vi "Report.vi"(4 "GuiRef":T1={"StringOut"=refnum, "AbortOnFail"=refnum, "SN"=refnum, "SN_Length"=refnum, "TestResult"=refnum, "Starttime"=refnum, "CycleTime"=refnum, "ErrorCode"=refnum, "UUTStatus"=refnum, "DataBaseEnable?"=refnum, "DUTModel"=refnum, "FixtureID"=refnum, "OperatorID"=refnum, "SNReady"=refnum, "StopSlot"=refnum, "NextStep"=refnum, "SlotStart?"=refnum, "PassYeild"=refnum, "Failed"=refnum, "Passed"=refnum, "Tested"=refnum, "ErrorStop"=refnum, "SlotReady"=refnum, "StartTest"=refnum, "TestItemsCtl"={"StepName"="", "TestEnable"=FALSE, "LoopCount"=0, "StopOnFail"=FALSE, "LastStep?"=FALSE, "Index"=0, "Para1"="", "Para2"="", "Para3"="", "Para4"="", "Para5"="", "TimeStart"=0}, "ProcessBar"=refnum, "Slot"=enum."Slot1", "Row"=3, "States"=refnum, "TestMode"=refnum, "PassYeild"=refnum, "ShowSkipStep?"=FALSE, "IniConfig"=refnum, "循环次数-DUT"=refnum, "开始按钮-DUT"=refnum, "选择方式"=refnum, "ExcelNames"=refnum, "TestPara"=refnum, "DAQmx设备名"=refnum, "波形图"=refnum, "调试模式"=refnum, "输入电压"=refnum, "产品型号"=refnum, "上电"=refnum, "测试结果"=refnum, "测试项目"=refnum, "DAQConfig"=refnum}, 5 "Report":string[][](array[string]), 6 "TestConfig":string[][](array[string]), 7 "索引":i32=2, 8 "index":i32=3, 9 "FailStep":string="XXX", 10 "TestResult":bool, 11 "TestStep":string="小灯") -> (3 "ReportOut":string[][](array[string]))   [LabVIEW 2013]
uses:
  SystemCode/Subvi/RefToString.vi
  <vilib>/Utility/miscctls.llb/LVRowAndColumnUnsignedTypeDef.ctl
  SystemCode/SysControl/TestItemsCTL.ctl
  SystemCode/SysControl/Slot.ctl
  SystemCode/SysControl/Reference.ctl
panel:
  out "StepReport":string[](array[string])
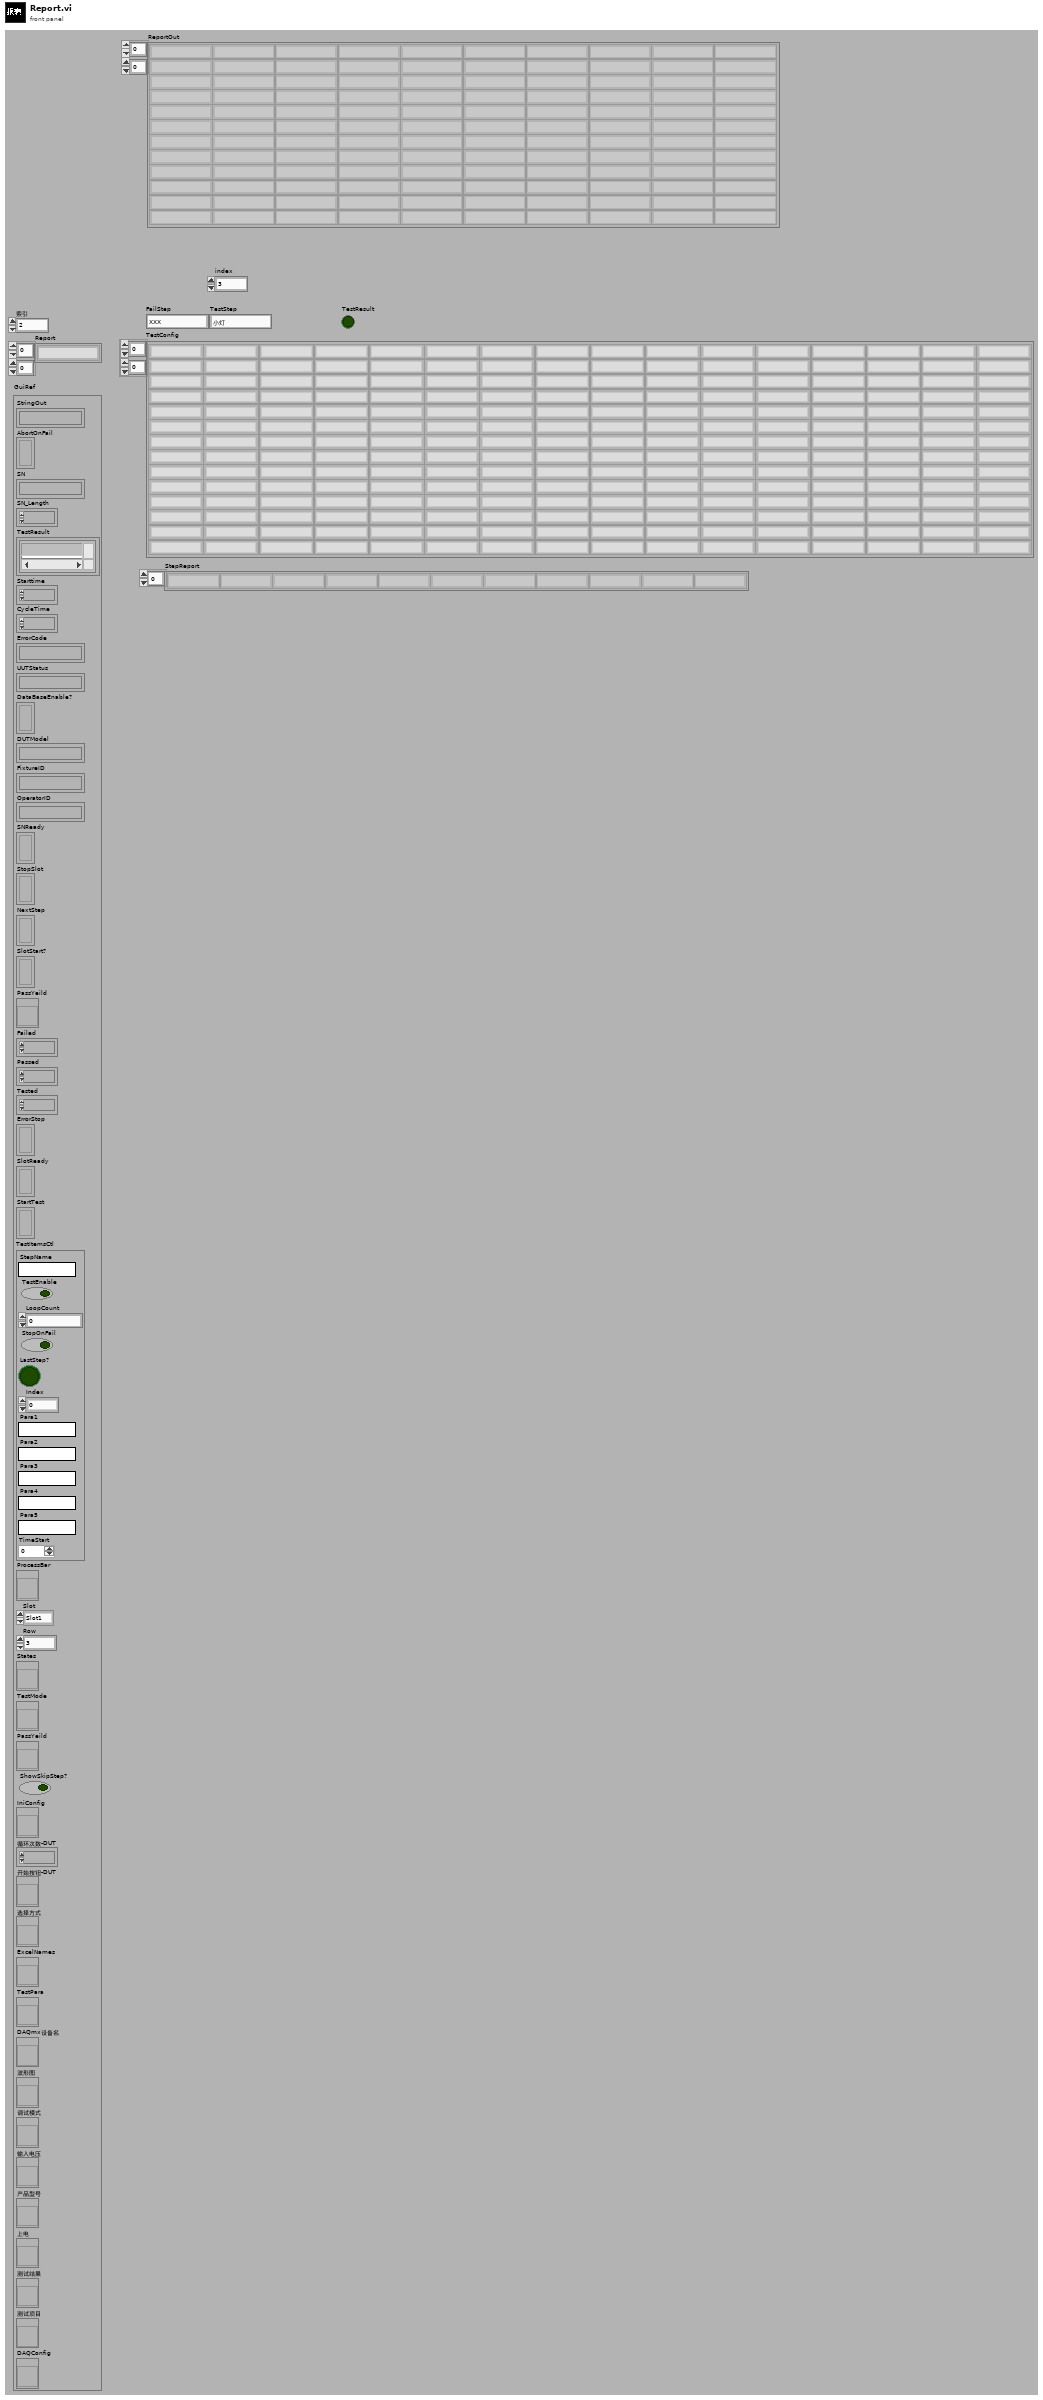
[diagram p1: front panel]
types:
  T1 = typedef "Reference.ctl" = cluster{"StringOut":refnum<vi>, "AbortOnFail":refnum<vi>, "SN":refnum<vi>, "SN_Length":refnum<vi>, "TestResult":refnum<vi>, "Starttime":refnum<vi>, "CycleTime":refnum<vi>, "ErrorCode":refnum<vi>, "UUTStatus":refnum<vi>, "DataBaseEnable?":refnum<vi>, "DUTModel":refnum<vi>, "FixtureID":refnum<vi>, "OperatorID":refnum<vi>, "SNReady":refnum<vi>, "StopSlot":refnum<vi>, "NextStep":refnum<vi>, "SlotStart?":refnum<vi>, "PassYeild":refnum<vi>, "Failed":refnum<vi>, "Passed":refnum<vi>, "Tested":refnum<vi>, "ErrorStop":refnum<vi>, "SlotReady":refnum<vi>, "StartTest":refnum<vi>, "TestItemsCtl":T2, "ProcessBar":refnum<vi>, "Slot":T3, "Row":i32, "States":refnum<vi>, "TestMode":refnum<vi>, "PassYeild":refnum<vi>, "ShowSkipStep?":bool, "IniConfig":refnum<vi>, "循环次数-DUT":refnum<vi>, "开始按钮-DUT":refnum<vi>, "选择方式":refnum<vi>, "ExcelNames":refnum<vi>, "TestPara":refnum<vi>, "DAQmx设备名":refnum<vi>, "波形图":refnum<vi>, "调试模式":refnum<vi>, "输入电压":refnum<vi>, "产品型号":refnum<vi>, "上电":refnum<vi>, "测试结果":refnum<vi>, "测试项目":refnum<vi>, "DAQConfig":refnum<vi>}
  T2 = typedef "TestItemsCTL.ctl" = cluster{"StepName":string, "TestEnable":bool, "LoopCount":i32, "StopOnFail":bool, "LastStep?":bool, "Index":i32, "Para1":string, "Para2":string, "Para3":string, "Para4":string, "Para5":string, "TimeStart":u32}
  T3 = typedef "Slot.ctl" = enum16{"Slot1", "Slot2", "Slot3", "Slot4"}
  T4 = typedef "LVRowAndColumnUnsignedTypeDef.ctl" = cluster{"Row":u32, "Column":u32}
  T5 = enum32{"invalid app kind", "Development System", "Run Time System", "Student Edition", "Embedded LabVIEW", "Evaluation", "Custom"}
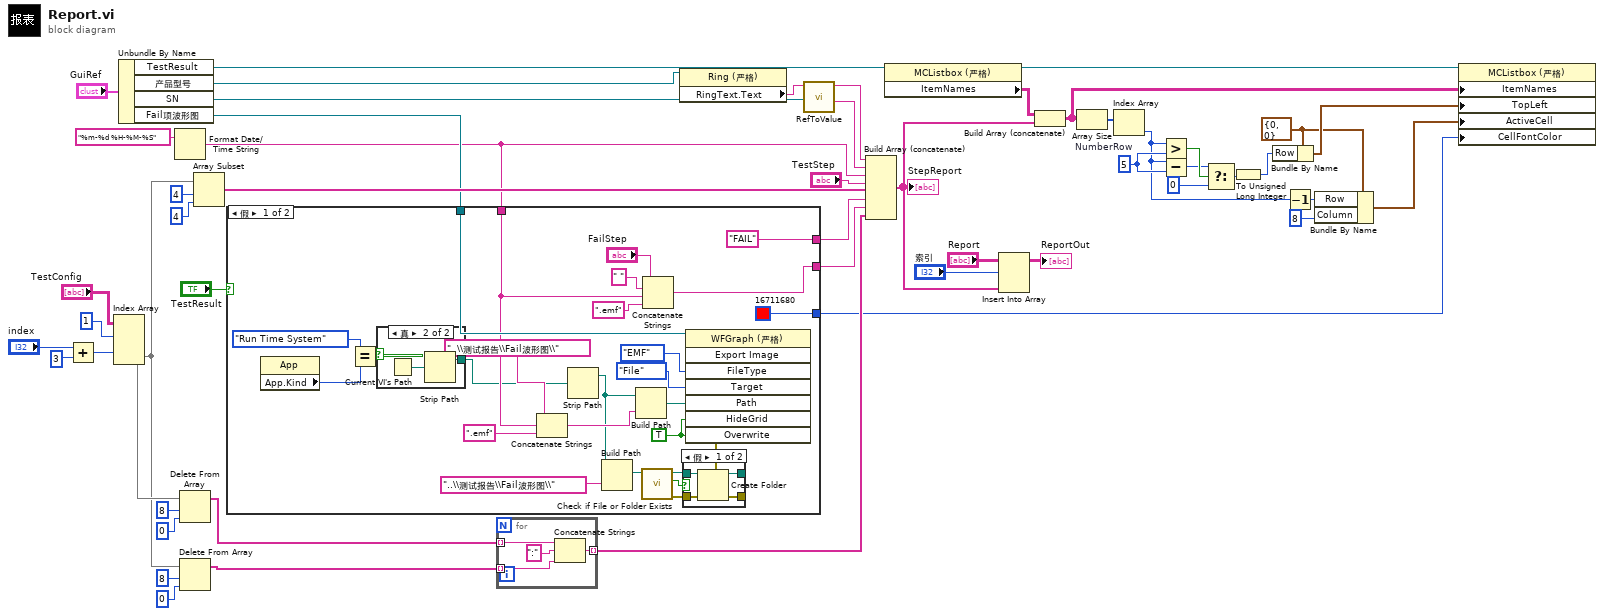
[diagram p0: block diagram]
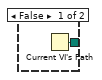
[diagram p3: hidden frame]
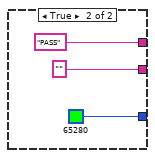
[diagram p4: hidden frame]
diagram:
  w4 = T4 {"Row"=0, "Column"=0} ("Top Left Visible Cell")
  w28 = 5  # NumberRow
  n1 = Add(x="index", y=3) -> (x+y=w33:i32)
  n2 = Index Array(array="TestConfig", index (row) #1=1 ("索引 (行)"), index (row) #2=w33) -> (element #1=w47:string[], element #2=w19:string[])  [unwired: 2 in]
  n3 = Unbundle By Name("GuiRef") -> ("TestResult"=w16:refnum<vi>, "产品型号"=w10:refnum<vi>, "SN"=w31:refnum<vi>, "Fail项波形图"=w18:refnum<vi>)
  n4 = Format Date/Time String(time format string (%c)="%m-%d %H-%M-%S" ("时间格式字符串(%c)")) -> (date/time string=w17:string)  [unwired: 2 in]
  n5 = Delete From Array(array=w47, length=8 ("长度"), index=0 ("索引")) -> (array with subset deleted=w46:string[])  [unwired: 1 out]
  n6 = Delete From Array(array=w19, length=8 ("长度"), index=0 ("索引")) -> (array with subset deleted=w45:string[])  [unwired: 1 out]
  n7 = Array Subset(array=w19, index=4 ("索引"), length=4 ("长度")) -> (w40:string[])
  n8 = case shown="假" "TestResult" {
    tunnel: ["FAIL" ("元素") "PASS" ("元素")] -> w37
    tunnel: [w67 "" ("FailStep")] -> w36
    tunnel: w18 -> [w72 _]
    tunnel: w17 -> [w68 _]
    tunnel: [u32 16711680 u32 65280] -> w5
    frame False {
      w73 = TRUE ("始终覆盖")
      n9 = property class="App"() -> ("App.Kind"=w62:T5)  [unwired: 2 in, 2 out]
      n10 = Equal?(x=T5."Run Time System" ("y"), y=w62) -> (x = y?=w61:bool)
      n11 = case shown="真" w61 {
        tunnel: [w83 w85] -> w60
        frame False {
          n12 = Current VI's Path() -> (path=w83:path)
        }
        frame True {
          n13 = Current VI's Path() -> (path=w84:path)
          n14 = Strip Path(path=w84) -> (stripped path=w85:path)  [unwired: 1 out]
        }
      }
      n15 = Concatenate Strings("..\\测试报告\\Fail波形图\\" ("字符串"), w68, ".emf" ("字符串")) -> (w65:string)
      n16 = Strip Path(path=w60) -> (stripped path=w58:path)  [unwired: 1 out]
      n17 = Build Path(base path=w58, name or relative path="..\\测试报告\\Fail波形图\\" ("字符串")) -> (appended path=w57:path)
      n18 = Build Path(base path=w58, name or relative path=w65) -> (appended path=w64:path)
      n19 = call <vilib>:"Check if File or Folder Exists.vi"("path"=w57) -> ("error out"=w54:errorcluster, "file or folder exists?"=w55:bool, "dup path"=w56:path)  [unwired: 1 in, 7 out]
      n20 = Concatenate Strings("FailStep", " " ("字符串"), w68, ".emf" ("字符串")) -> (w67:string)
      n21 = case shown="假" w55 {
        tunnel: w56 -> [w81 w82]
        tunnel: [w80 _] -> w53
        tunnel: w54 -> [w79 _]
        tunnel: [w78 w82] -> _
        frame False {
          n22 = Create Folder(path (use dialog)=w81, error in=w79) -> (created path=w78:path, error out=w80:errorcluster)  [unwired: 2 out]
        }
        frame True {
        }
      }
      n23 = invoke on="调用节点" class="WFGraph (严格)" method="Export Image"(reference=w72, error in=w53, "FileType"=enum32{"BMP", "EPS", "EMF", "PICT"}."EMF" ("文件类型"), "Target"=enum32{"File", "Clipboard"}."File" ("终端"), "Path"=w64, "HideGrid"=w73, "Overwrite"=w73) -> ()  [unwired: 1 in, 8 out]
    }
    frame True {
    }
  }
  n24 = for {
    tunnel: w46 -> [w92] mode=indexing
    tunnel: w45 -> [w91] mode=indexing
    tunnel: [w89] -> w39 mode=indexing
    n25 = Concatenate Strings(w92, ":" ("字符串"), w91) -> (w89:string)
  }
  n26 = property class="Ring (严格)"(reference=w10) -> ("RingText.Text"=w9:string)  [unwired: 1 in, 2 out]
  n27 = call-poly "RefToValue.vi"("StrRef"=w31) -> ("String"=w30:string)  [unwired: 5 in, 1 out]
  n28 = Build Array (concatenate)(w9, w30, w17, "TestStep", w40, w37, w36, w39) -> (w13:string[])
  "StepReport" <- w13
  n29 = property class="MCListbox (严格)"(reference=w16) -> (reference out=w11:refnum<vi>, "ItemNames"=w14:string[][])  [unwired: 1 in, 1 out]
  n30 = Insert Into Array(array="Report", index (row)="索引", new element=w13) -> (→"ReportOut":string[][])  [unwired: 1 in]
  n31 = Build Array (concatenate)(w14, w13) -> (w12:string[][])
  n32 = Array Size(array=w12) -> (size(s)=w23:i32[])
  n33 = Index Array(array=w23) -> (element=w1:i32)  [unwired: 1 in]
  n34 = Greater?(x=w1, y=w28) -> (0:w27:bool)
  n35 = Subtract(x=w1, y=w28) -> (x-y=w25:i32)
  n36 = Select(t=w25, s=w27, f=0) -> (s? t:f=w24:i32)
  n37 = To Unsigned Long Integer(number=w24) -> (unsigned 32bit integer=w29:u32)
  n38 = Bundle By Name(cluster=w4, "Row"=w29) -> (w8:T4)
  n39 = Decrement(x=w1) -> (x-1=w2:i32)
  n40 = Bundle By Name(cluster=w4, "Row"=w2, "Column"=u32 8) -> (w6:T4)
  n41 = property class="MCListbox (严格)"(reference=w11, "ItemNames"=w12, "TopLeft"=w8, "ActiveCell"=w6, "CellFontColor"=w5) -> ()  [unwired: 1 in, 2 out]
